vi "DialogCreateClass_ReadTemplatesFilterSettings.vi"(11 "AllTemplatesForThisProvider/InheritanceType(Base/Sub)":T1[](array[typedef])) -> (2 "FilterSettings(OrderIndex,Active)":cluster{"Numeric":i32, "Checkbox":bool}[](array[cluster]), 3 "Section":string)   [LabVIEW 2020, in "ClassWriterNative.lvclass"]
uses:
  <resource>/Framework/Providers/Open_GDS/ClassProviders/Provider_LvNativeClass/ClassWriterNative_class/ClassWriterNative.lvclass
  <resource>/Framework/Providers/Open_GDS/ClassProviders/Provider_BaseClassInterface/ClassTemplateType.ctl
  <vilib>/Utility/config.llb/Read Key (String).vi
  <vilib>/Utility/config.llb/NI_LVConfig.lvlib
  <resource>/Framework/Providers/Open_GDS/ClassProviders/Provider_BaseClassInterface/ClassWriter_class/ClassWriter.lvclass
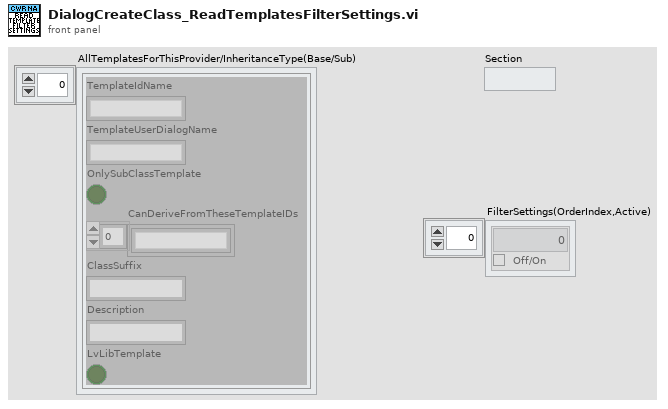
[diagram p1: front panel]
types:
  T1 = typedef "ClassWriter.lvclass/ClassTemplateType.ctl" = cluster{"TemplateIdName":string, "TemplateUserDialogName":string, "OnlySubClassTemplate":bool, "CanDeriveFromTheseTemplateIDs":string[], "ClassSuffix":string, "Description":string, "LvLibTemplate":bool}
  T2 = typedef "NI_LVConfig.lvlib/Config Data RefNum.ctl" = refnum<k1>
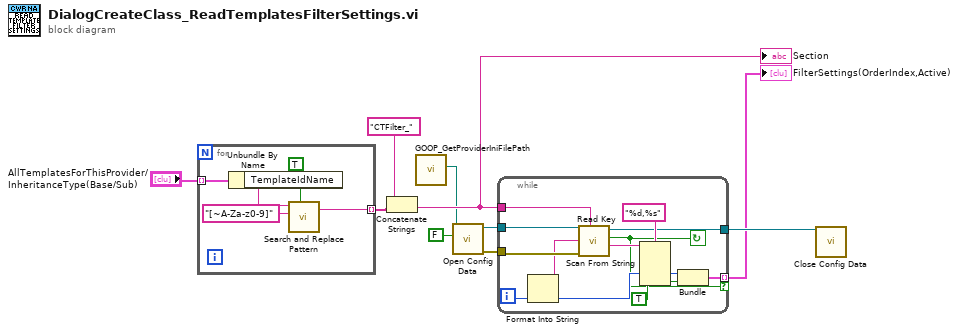
[diagram p0: block diagram]
diagram:
  n1 = for {
    tunnel: "AllTemplatesForThisProvider/InheritanceType(Base/Sub)" -> [w15] mode=indexing
    tunnel: [w11] -> w2 mode=indexing
    n2 = Unbundle By Name(w15) -> ("TemplateIdName"=w14:string)
    n3 = call <vilib>:"Search and Replace Pattern.vi"("string"=w14, "regular expression (\"\")"="[~A-Za-z0-9]" ("regular expression (\"\")"), "replace all? (F)"=TRUE) -> ("result string"=w11:string)  [unwired: 2 in, 1 out]
  }
  n4 = Concatenate Strings("CTFilter_" ("regular expression (\"\")"), w2) -> (w10:string)
  "Section" <- w10
  n5 = call <resource>:"GOOP_GetProviderIniFilePath.vi"() -> ("ProviderIniPath"=w3:path)  [unwired: 10 in, 1 out]
  n6 = call <vilib>:"Open Config Data.vi"("create file if necessary (T)"=FALSE, "configuration file path"=w3) -> ("error out"=w6:errorcluster, "refnum"=w5:T2)  [unwired: 7 in, 1 out]
  n7 = while {
    tunnel: w5 -> [w28]
    tunnel: w6 -> [w27]
    tunnel: w10 -> [w26]
    tunnel: [w18] -> w7 mode=indexing if=w17
    tunnel: [w16] -> w8
    i -> [w22]
    stop <- w17 continue-if-true
    n8 = Format Into String(w22) -> (resulting string=w25:string)  [unwired: 3 in, 1 out]
    n9 = call-poly <vilib>:"Read Key.vi"("section"=w26, "error in (no error)"=w27, "key"=w25, "refnum"=w28) -> ("value"=w24:string, "found?"=w17:bool, "refnum out"=w16:T2)  [unwired: 4 in, 1 out]
    n10 = Scan From String(format string="%d,%s", input string=w24, default 1=w22, default 2=TRUE) -> (output 1=w20:i32, output 2=w19:bool)  [unwired: 2 in, 3 out]
    n11 = Bundle(w20, w19) -> (w18:cluster{i32, bool})  [unwired: 1 in]
  }
  "FilterSettings(OrderIndex,Active)" <- w7
  n12 = call <vilib>:"Close Config Data.vi"("refnum"=w8) -> ()  [unwired: 9 in, 2 out]
